vi "FuncImg-Initialisation.vi"(6 "Functional Imging UI Refs":T1) -> ()   [LabVIEW 2013]
uses:
  Typedefs/Functional Imging UI Refs.ctl
  xcontrol/XGrapher.xctl
  Typedefs/ROI selector array-ROI vis.ctl
  xcontrol/Interface VIs/Interface typedefs/Interface-ROI selection cluster.ctl
  Typedefs/ROI ID Enum.ctl
  Typedefs/Groups array referecne.ctl
  Typedefs/ROI visibility mode.ctl
  Global variables/gl_Functional Imaging-Global variables.vi
panel:
  # "[Groups] is a Typedef"
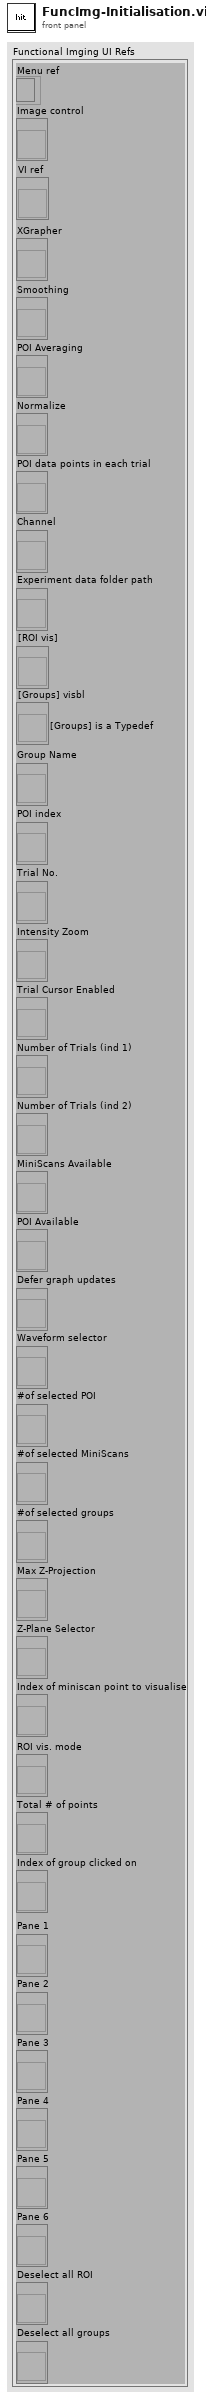
[diagram p1: front panel]
types:
  T1 = typedef "Functional Imging UI Refs.ctl" = cluster{"Menu ref":refnum<k9>, "Image control":refnum<vi>, "VI ref":refnum<vi>, "XGrapher":refnum<vi>, "Smoothing":refnum<vi>, "POI Averaging":refnum<vi>, "Normalize":refnum<vi>, "POI data points in each trial":refnum<vi>, "Channel":refnum<vi>, "Experiment data folder path":refnum<vi>, "[ROI vis]":refnum<vi>, "[Groups] visbl":T2, "Group Name":refnum<vi>, "POI index":refnum<vi>, "Trial No.":refnum<vi>, "Intensity Zoom":refnum<vi>, "Trial Cursor Enabled":refnum<vi>, "Number of Trials (ind 1)":refnum<vi>, "Number of Trials (ind 2)":refnum<vi>, "MiniScans Available":refnum<vi>, "POI Available":refnum<vi>, "Defer graph updates":refnum<vi>, "Waveform selector":refnum<vi>, "#of selected POI":refnum<vi>, "#of selected MiniScans":refnum<vi>, "#of selected groups":refnum<vi>, "Max Z-Projection":refnum<vi>, "Z-Plane Selector":refnum<vi>, "Index of miniscan point to visualise":refnum<vi>, "ROI vis. mode":refnum<vi>, "Total # of points":refnum<vi>, "Index of group clicked on":refnum<vi>, "Pane 1":refnum<vi>, "Pane 2":refnum<vi>, "Pane 3":refnum<vi>, "Pane 4":refnum<vi>, "Pane 5":refnum<vi>, "Pane 6":refnum<vi>, "Deselect all ROI":refnum<vi>, "Deselect all groups":refnum<vi>}
  T2 = typedef "Groups array referecne.ctl" = refnum<vi>
  T3 = enum32{"Invalid", "Standard", "Closed", "Hidden", "Minimized", "Maximized"}
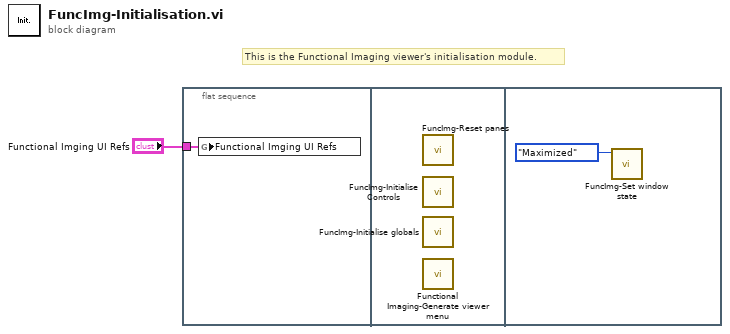
[diagram p0: block diagram]
diagram:
  # "This is the Functional Imaging viewer's initialisation module."
  n1 = flat-sequence {
    tunnel: "Functional Imging UI Refs" -> [w2]
    frame #0 {
      n2 = global write "gl_Functional Imaging-Global variables.vi" "Functional Imging UI Refs"(w2) -> ()
    }
    frame #1 {
      n3 = call "FuncImg-Reset panes.vi"() -> ()  [unwired: 12 in]
      n4 = call "FuncImg-Initialise Controls.vi"() -> ()  [unwired: 12 in]
      n5 = call "FuncImg-Initialise globals.vi"() -> ()  [unwired: 12 in]
      n6 = call "Functional Imaging-Generate viewer menu.vi"() -> ()  [unwired: 10 in, 2 out]
    }
    frame #2 {
      n7 = call "FuncImg-Set window state.vi"("Front Panel Window:State"=T3."Maximized") -> ()  [unwired: 10 in, 1 out]
    }
  }
